vi "LSMcontroller_v64_updatedwaveformhandling.vi"() -> ()   [LabVIEW 2015] (continued)
                                n1313 = case shown="False" w3862 {
                                tunnel: [w3868 w3888] -> w3861
                                tunnel: [w3867 FALSE ("removal")] -> w3860
                                tunnel: [w3866 w3886] -> w3859
                                tunnel: w3858 -> [w3865 _]
                                frame False {
                                n1314 = case shown="False" w3865 {
                                tunnel: [FALSE ("addition") FALSE ("addition")] -> w3868
                                tunnel: [w3870 FALSE ("removal")] -> w3867
                                tunnel: [w3869 _] -> w3866
                                frame False {
                                n1315 = call "configuration.vi"("command"="get") -> ("config out"=w3876:T11)  [unwired: 2 in, 1 out]
                                n1316 = Unbundle By Name(w3876) -> ("2P shutter"=w3873:i32)
                                n1317 = call "2pparameters.vi"("command"="get") -> ("params out"=w3874:T10)  [unwired: 1 in]
                                n1318 = in-place {
                                in-place-border: w3873 -> [w3883]
                                in-place-border: [w3880] -> w3870
                                in-place-border: [w3879] -> w3869
                                n1319 = in-place-cluster #25(w3874) -> ("aDO"=w3882:u32[])
                                n1320 = call "remove channel from active arrayv2.vi"("line array in"=w3882, "line to remove"=w3883) -> ("line array out"=w3881:u32[], "removal"=w3880:bool, "index"=w3879:i32)
                                n1321 = in-place-cluster #25("aDO"=w3881) -> (w3871:T10)
                                }
                                n1322 = call "2pparameters.vi"("Params in"=w3871, "command"="set") -> ()  [unwired: 1 out]
                                }
                                frame True {
                                }
                                }
                                }
                                frame True {
                                n1323 = call "configuration.vi"("command"="get") -> ("config out"=w3890:T11)  [unwired: 2 in, 1 out]
                                n1324 = call "2pparameters.vi"("command"="get") -> ("params out"=w3894:T10)  [unwired: 1 in]
                                n1325 = Unbundle By Name(w3890) -> ("2P shutter"=w3889:i32)
                                n1326 = in-place {
                                in-place-border: w3889 -> [w3900]
                                in-place-border: [w3897] -> w3888
                                in-place-border: [w3896] -> w3886
                                n1327 = in-place-cluster #26(w3894) -> ("aDO"=w3899:u32[])
                                n1328 = call "add channel to active arrayv2.vi"("line array in"=w3899, "line to add"=w3900) -> ("line array out"=w3898:u32[], "addition"=w3897:bool, "index"=w3896:i32)
                                n1329 = in-place-cluster #26("aDO"=w3898) -> (w3892:T10)
                                }
                                n1330 = call "2pparameters.vi"("Params in"=w3892, "command"="set") -> ()  [unwired: 1 out]
                                }
                                }
                                }
                                frame #3 {
                                n1331 = local read "Measurement"() -> (w3904:T4)
                                n1332 = To Unsigned Long Integer(number=w3904) -> (unsigned 32bit integer=w3905:u32)
                                n1333 = case shown="5..7" w3905 {
                                tunnel: [FALSE ("addition") w3923] -> w3903
                                tunnel: [w3908 FALSE ("removal")] -> w3902
                                tunnel: [w3906 w3921] -> w3901
                                frame 0..4, Default {
                                n1334 = call "configuration.vi"("command"="get") -> ("config out"=w3914:T11)  [unwired: 2 in, 1 out]
                                n1335 = Unbundle By Name(w3914) -> ("LT timestamp"=w3911:u32)
                                n1336 = call "2pparameters.vi"("command"="get") -> ("params out"=w3912:T10)  [unwired: 1 in]
                                n1337 = in-place {
                                in-place-border: w3911 -> [w3920]
                                in-place-border: [w3917] -> w3908
                                in-place-border: [w3916] -> w3906
                                n1338 = in-place-cluster #27(w3912) -> ("aDO"=w3919:u32[])
                                n1339 = call "remove channel from active arrayv2.vi"("line array in"=w3919, "line to remove"=w3920) -> ("line array out"=w3918:u32[], "removal"=w3917:bool, "index"=w3916:i32)
                                n1340 = in-place-cluster #27("aDO"=w3918) -> (w3909:T10)
                                }
                                n1341 = call "2pparameters.vi"("Params in"=w3909, "command"="set") -> ()  [unwired: 1 out]
                                }
                                frame 5..7 {
                                n1342 = call "configuration.vi"("command"="get") -> ("config out"=w3929:T11)  [unwired: 2 in, 1 out]
                                n1343 = Unbundle By Name(w3929) -> ("LT timestamp"=w3926:u32)
                                n1344 = call "2pparameters.vi"("command"="get") -> ("params out"=w3927:T10)  [unwired: 1 in]
                                n1345 = in-place {
                                in-place-border: w3926 -> [w3935]
                                in-place-border: [w3932] -> w3923
                                in-place-border: [w3931] -> w3921
                                n1346 = in-place-cluster #28(w3927) -> ("aDO"=w3934:u32[])
                                n1347 = call "add channel to active arrayv2.vi"("line array in"=w3934, "line to add"=w3935) -> ("line array out"=w3933:u32[], "addition"=w3932:bool, "index"=w3931:i32)
                                n1348 = in-place-cluster #28("aDO"=w3933) -> (w3924:T10)
                                }
                                n1349 = call "2pparameters.vi"("Params in"=w3924, "command"="set") -> ()  [unwired: 1 out]
                                }
                                }
                                }
                                }
                                }
                                frame #1 {
                                n1350 = Or(x=w3942, y=w3943) -> (x .or. y?=w3941:bool)
                                n1351 = case shown="True" w3941 {
                                frame False {
                                }
                                frame True {
                                # "update GUI"
                                n1352 = call "Used AO lines.vi"() -> ("used AO names"=w3947:string[], "used AO lines"=w3949:tag[])  [unwired: 2 in]
                                n1353 = control-ref of="Analog Lines Plot"() -> (w3948:refnum<vi>)
                                n1354 = local write "Analog Used Lines"(w3949) -> ()
                                n1355 = local write "Analog Used Names"(w3947) -> ()
                                n1356 = call "prepAOWaveplot.vi"("WaveformGraph in"=w3948, "Analog Used Names"=w3947) -> ()  [unwired: 1 in]
                                }
                                }
                                n1357 = Compound Arithmetic op=OR(w3939, w3938, w3937, w3936) -> (w3940:bool)
                                n1358 = case shown="True" w3940 {
                                frame False {
                                }
                                frame True {
                                n1359 = control-ref of="Digital Lines Plot"() -> (w3944:refnum<vi>)
                                n1360 = call "Used DO lines.vi"() -> ("used DO names"=w3945:string[], "used DO lines"=w3946:tag[])  [unwired: 2 in]
                                n1361 = local write "Digital Used Lines"(w3946) -> ()
                                n1362 = local write "Digital Used Names"(w3945) -> ()
                                n1363 = call "prepDOWaveplot.vi"("DigitalGraph in"=w3944, "used DO names"=w3945) -> ()  [unwired: 1 in]
                                }
                                }
                                }
                                frame #2 {
                                n1364 = case shown="False" w3953 {
                                tunnel: [w3956 w3982] -> w3952
                                tunnel: [w3955 w3980] -> w3951
                                tunnel: [w3954 _] -> w3950
                                frame False {
                                n1365 = stacked-sequence {
                                seq-local: [w3958 _] -> [_ w3973]
                                tunnel: [w3958 _] -> w3956
                                tunnel: [w3961 _] -> w3955
                                tunnel: [w3957 _] -> w3954
                                frame #0 {
                                n1366 = call "configuration.vi"("command"="get") -> ("config out"=w3969:T11)  [unwired: 2 in, 1 out]
                                n1367 = call "waveformparamsv2.vi"("command"="get") -> ("Params out"=w3963:T14)  [unwired: 4 in, 2 out]
                                n1368 = Unbundle By Name(w3969) -> ("Voltage to Xgalvo"=w3970:i32)
                                n1369 = call "2pparameters.vi"("command"="get") -> ("params out"=w3966:T10)  [unwired: 1 in]
                                n1370 = Unbundle By Name(w3963) -> ("AO parameters"=w3962:T15)
                                n1371 = Unbundle By Name(w3966) -> ("aAO"=w3967:u32[])
                                n1372 = call "waveformsAObuffer.vi"("command"="get") -> ("AO wf out"=w3959:waveform(dbl)[])  [unwired: 1 in]
                                n1373 = Search 1D Array(1D array=w3967, element=w3970) -> (index of element=w3958:i32)  [unwired: 1 in]
                                n1374 = Index Array(array=w3959, index=w3958) -> (element=w3957:waveform(dbl))
                                n1375 = Index Array(array=w3962, index=w3958) -> (element=w3961:T16)
                                }
                                frame #1 {
                                w3974 = 0.0 ("Step size (V)")
                                n1376 = local read "Meastab"() -> (w3972:enum32{"X-Y Image", "Linescan", "Timetrace"})
                                n1377 = case shown="\"X-Y Image\", Default" w3972 {
                                tunnel: [w3976 w3977] -> w3971
                                frame "X-Y Image", Default {
                                n1378 = local read "Sampling rate"() -> (w3976:dbl)
                                }
                                frame "Timetrace" {
                                n1379 = local read "srateAODOtt"() -> (w3977:dbl)
                                }
                                }
                                n1380 = call "replace AO XYwfparam.vi"("Baseline (V)"=w3974, "Start amplitude (V)"=w3974, "Cycles"=w3974, "Repeats"=w3974, "index of AO wave"=w3973, "Step size (V)"=w3974, "DC (%)"=w3974, "Sampling frequency (Hz)"=w3971, "Period (ms)"=w3974, "Cycle length (s)"=w3974, "Pulses"=w3974, "padding value"=w3974, "Matlab wave name"=path "xwave") -> ()  [unwired: 3 in]
                                }
                                }
                                }
                                frame True {
                                w3981 = 0.0 ("Repeats")
                                n1381 = local read "Meastab"() -> (w3979:enum32{"X-Y Image", "Linescan", "Timetrace"})
                                n1382 = case shown="\"X-Y Image\", Default" w3979 {
                                tunnel: [w3998 w3999] -> w3978
                                frame "X-Y Image", Default {
                                n1383 = local read "Sampling rate"() -> (w3998:dbl)
                                }
                                frame "Timetrace" {
                                n1384 = local read "srateAODOtt"() -> (w3999:dbl)
                                }
                                }
                                n1385 = call "2pparameters.vi"("command"="get") -> ("params out"=w3984:T10)  [unwired: 1 in]
                                n1386 = call "configuration.vi"("command"="get") -> ("config out"=w3987:T11)  [unwired: 2 in, 1 out]
                                n1387 = call "waveformparamsv2.vi"("command"="get") -> ("Params out"=w3995:T14)  [unwired: 4 in, 2 out]
                                n1388 = Unbundle By Name(w3987) -> ("Voltage to Xgalvo"=w3988:i32)
                                n1389 = Unbundle By Name(w3995) -> ("AO parameters"=w3992:T15)
                                n1390 = Unbundle By Name(w3984) -> ("aAO"=w3985:u32[])
                                n1391 = Search 1D Array(1D array=w3985, element=w3988) -> (index of element=w3982:i32)  [unwired: 1 in]
                                n1392 = Index Array(array=w3992, index=0) -> (element=w3993:T16)
                                n1393 = Bundle By Name(cluster=w3993, "AOtab"=-1.0 ("Repeats"), "Repeats"=w3981, "Cycles"=w3981, "Start amplitude (V)"=w3981, "Baseline (V)"=w3981, "Step size (V)"=w3981, "DC (%)"=w3981, "Sampling frequency (Hz)"=w3978, "Period (ms)"=w3981, "Offset (V)"=w3981, "Amplitude (V)"=w3981, "Frequency"=w3981, "Tri Repeats"=w3981, "phase shift (ms)"=w3981, "Pulses"=w3981, "Matlab wave file"=path "xwave", "padding value"=w3981) -> (w3980:T16)
                                n1394 = Build Array(w3980) -> (w3990:T15)
                                n1395 = call "waveformparamsv2.vi"("command"="add AO", "add AO"=w3990) -> ()  [unwired: 3 in, 3 out]
                                }
                                }
                                }
                                frame #3 {
                                n1396 = case shown="False" w4003 {
                                tunnel: [w4006 w4032] -> w4002
                                tunnel: [w4005 w4030] -> w4001
                                tunnel: [w4004 _] -> w4000
                                frame False {
                                n1397 = stacked-sequence {
                                seq-local: [w4008 _] -> [_ w4023]
                                tunnel: [w4008 _] -> w4006
                                tunnel: [w4011 _] -> w4005
                                tunnel: [w4007 _] -> w4004
                                frame #0 {
                                n1398 = call "configuration.vi"("command"="get") -> ("config out"=w4019:T11)  [unwired: 2 in, 1 out]
                                n1399 = call "waveformparamsv2.vi"("command"="get") -> ("Params out"=w4013:T14)  [unwired: 4 in, 2 out]
                                n1400 = Unbundle By Name(w4019) -> ("Voltage to Ygalvo"=w4020:i32)
                                n1401 = call "2pparameters.vi"("command"="get") -> ("params out"=w4016:T10)  [unwired: 1 in]
                                n1402 = Unbundle By Name(w4013) -> ("AO parameters"=w4012:T15)
                                n1403 = Unbundle By Name(w4016) -> ("aAO"=w4017:u32[])
                                n1404 = call "waveformsAObuffer.vi"("command"="get") -> ("AO wf out"=w4009:waveform(dbl)[])  [unwired: 1 in]
                                n1405 = Search 1D Array(1D array=w4017, element=w4020) -> (index of element=w4008:i32)  [unwired: 1 in]
                                n1406 = Index Array(array=w4009, index=w4008) -> (element=w4007:waveform(dbl))
                                n1407 = Index Array(array=w4012, index=w4008) -> (element=w4011:T16)
                                }
                                frame #1 {
                                w4024 = 0.0 ("Step size (V)")
                                n1408 = local read "Meastab"() -> (w4022:enum32{"X-Y Image", "Linescan", "Timetrace"})
                                n1409 = case shown="\"X-Y Image\", Default" w4022 {
                                tunnel: [w4026 w4027] -> w4021
                                frame "X-Y Image", Default {
                                n1410 = local read "Sampling rate"() -> (w4026:dbl)
                                }
                                frame "Timetrace" {
                                n1411 = local read "srateAODOtt"() -> (w4027:dbl)
                                }
                                }
                                n1412 = call "replace AO XYwfparam.vi"("Baseline (V)"=w4024, "Start amplitude (V)"=w4024, "Cycles"=w4024, "Repeats"=w4024, "index of AO wave"=w4023, "Step size (V)"=w4024, "DC (%)"=w4024, "Sampling frequency (Hz)"=w4021, "Period (ms)"=w4024, "Cycle length (s)"=w4024, "Pulses"=w4024, "padding value"=w4024, "Matlab wave name"=path "ywave") -> ()  [unwired: 3 in]
                                }
                                }
                                }
                                frame True {
                                w4031 = 0.0 ("Repeats")
                                n1413 = local read "Meastab"() -> (w4029:enum32{"X-Y Image", "Linescan", "Timetrace"})
                                n1414 = case shown="\"X-Y Image\", Default" w4029 {
                                tunnel: [w4048 w4049] -> w4028
                                frame "X-Y Image", Default {
                                n1415 = local read "Sampling rate"() -> (w4048:dbl)
                                }
                                frame "Timetrace" {
                                n1416 = local read "srateAODOtt"() -> (w4049:dbl)
                                }
                                }
                                n1417 = call "2pparameters.vi"("command"="get") -> ("params out"=w4034:T10)  [unwired: 1 in]
                                n1418 = call "configuration.vi"("command"="get") -> ("config out"=w4037:T11)  [unwired: 2 in, 1 out]
                                n1419 = call "waveformparamsv2.vi"("command"="get") -> ("Params out"=w4046:T14)  [unwired: 4 in, 2 out]
                                n1420 = Unbundle By Name(w4037) -> ("Voltage to Ygalvo"=w4038:i32)
                                n1421 = Unbundle By Name(w4046) -> ("AO parameters"=w4043:T15)
                                n1422 = Unbundle By Name(w4034) -> ("aAO"=w4035:u32[])
                                n1423 = Search 1D Array(1D array=w4035, element=w4038) -> (index of element=w4032:i32)  [unwired: 1 in]
                                n1424 = Index Array(array=w4043, index=0) -> (element=w4044:T16)
                                n1425 = Bundle By Name(cluster=w4044, "AOtab"=-1.0 ("Repeats"), "Repeats"=w4031, "Cycles"=w4031, "Start amplitude (V)"=w4031, "Baseline (V)"=w4031, "Step size (V)"=w4031, "DC (%)"=w4031, "Sampling frequency (Hz)"=w4028, "Period (ms)"=w4031, "Offset (V)"=w4031, "Amplitude (V)"=w4031, "Frequency"=w4031, "Tri Repeats"=w4031, "phase shift (ms)"=w4031, "Pulses"=w4031, "Matlab wave file"=path "ywave", "padding value"=w4031) -> (w4030:T16)
                                n1426 = Build Array(w4030) -> (w4041:T15)
                                n1427 = call "waveformparamsv2.vi"("command"="add AO", "add AO"=w4041) -> ()  [unwired: 3 in, 3 out]
                                }
                                }
                                }
                                frame #4 {
                                n1428 = call "2pparameters.vi"("command"="get") -> ("params out"=w4055:T10)  [unwired: 1 in]
                                n1429 = Unbundle By Name(w4055) -> ("wavdet"=w4054:bool, "Pel"=w4051:sgl, "refwfsize"=w4050:dbl, "srateAODO"=w4053:sgl)
                                n1430 = case shown="True" w4054 {
                                tunnel: [w4059 w4069] -> w4057
                                tunnel: w4053 -> [w4060 w4071]
                                tunnel: w4051 -> [_ w4067]
                                tunnel: w4050 -> [_ w4066]
                                frame False {
                                n1431 = call "X-array-databuffer.vi"("command"=enum16{"get", "set", "clear", "append"}."get") -> ("array out"=w4063:dbl[])  [unwired: 3 in, 1 out]
                                n1432 = Reciprocal(x=w4060) -> (1/x=w4061:sgl)
                                n1433 = Bundle By Name("Y"=w4063, "dt"=w4061) -> (w4059:waveform(dbl))  [unwired: 1 in]
                                }
                                frame True {
                                n1434 = To Double Precision Float(number=w4067) -> (double precision float=w4068:dbl)
                                n1435 = Divide(x=w4066, y=w4068) -> (x/y=w4065:dbl)
                                n1436 = Round Toward +Infinity(x=w4065) -> (ceil(x): smallest int >= x=w4064:dbl)
                                n1437 = call "X-array-databuffer.vi"("command"=enum16{"get", "set", "clear", "append"}."get") -> ("array out"=w4073:dbl[])  [unwired: 3 in, 1 out]
                                n1438 = Reciprocal(x=w4071) -> (1/x=w4072:sgl)
                                n1439 = for {
                                N: w4064 -> [_]
                                tunnel: w4073 -> [w4075]
                                tunnel: [w4075] -> w4070 mode=concatenating
                                }
                                n1440 = Bundle By Name("Y"=w4070, "dt"=w4072) -> (w4069:waveform(dbl))  [unwired: 1 in]
                                }
                                }
                                n1441 = case shown="True" w4058 {
                                tunnel: w4057 -> [w4077 w4083]
                                tunnel: w4052 -> [w4078 _]
                                frame False {
                                n1442 = call "waveformsAObuffer.vi"("command"="get") -> ("AO wf out"=w4081:waveform(dbl)[])  [unwired: 1 in]
                                n1443 = property on="refwf" class="Ring (strict)" props=["RingText", "Text"]() -> ()  [unwired: 2 in, 3 out]
                                n1444 = Replace Array Subset(array=w4081, new element=w4077, index=w4078) -> (w4076:waveform(dbl)[])
                                n1445 = call "waveformsAObuffer.vi"("AO wf in"=w4076, "command"="set") -> ()  [unwired: 1 out]
                                }
                                frame True {
                                n1446 = call "waveformsAObuffer.vi"("command"="get") -> ("AO wf out"=w4085:waveform(dbl)[])  [unwired: 1 in]
                                n1447 = Build Array (concatenate)(w4085, w4083) -> (w4082:waveform(dbl)[])
                                n1448 = call "waveformsAObuffer.vi"("AO wf in"=w4082, "command"="set") -> ()  [unwired: 1 out]
                                }
                                }
                                }
                                frame #5 {
                                n1449 = call "2pparameters.vi"("command"="get") -> ("params out"=w4097:T10)  [unwired: 1 in]
                                n1450 = Unbundle By Name(w4097) -> ("wavdet"=w4096:bool, "Pel"=w4094:sgl, "refwfsize"=w4095:dbl, "srateAODO"=w4090:sgl)
                                n1451 = To Double Precision Float(number=w4094) -> (double precision float=w4093:dbl)
                                n1452 = Divide(x=w4095, y=w4093) -> (x/y=w4092:dbl)
                                n1453 = Round Toward +Infinity(x=w4092) -> (ceil(x): smallest int >= x=w4091:dbl)
                                n1454 = case shown="True" w4096 {
                                tunnel: [w4101 w4107] -> w4087
                                tunnel: w4091 -> [_ w4104]
                                tunnel: w4090 -> [w4102 w4109]
                                frame False {
                                n1455 = call "Y-array-databuffer.vi"("command"=enum16{"get", "set", "clear", "append"}."get") -> ("array out"=w4099:dbl[])  [unwired: 3 in, 1 out]
                                n1456 = Reciprocal(x=w4102) -> (1/x=w4103:sgl)
                                n1457 = Bundle By Name("Y"=w4099, "dt"=w4103) -> (w4101:waveform(dbl))  [unwired: 1 in]
                                }
                                frame True {
                                n1458 = call "Y-array-databuffer.vi"("command"=enum16{"get", "set", "clear", "append"}."get") -> ("array out"=w4105:dbl[])  [unwired: 3 in, 1 out]
                                n1459 = Reciprocal(x=w4109) -> (1/x=w4110:sgl)
                                n1460 = for {
                                N: w4104 -> [_]
                                tunnel: w4105 -> [w4111]
                                tunnel: [w4111] -> w4108 mode=concatenating
                                }
                                n1461 = Bundle By Name("Y"=w4108, "dt"=w4110) -> (w4107:waveform(dbl))  [unwired: 1 in]
                                }
                                }
                                n1462 = case shown="False" w4089 {
                                tunnel: w4087 -> [w4114 w4119]
                                tunnel: w4088 -> [w4115 _]
                                frame False {
                                n1463 = call "waveformsAObuffer.vi"("command"="get") -> ("AO wf out"=w4117:waveform(dbl)[])  [unwired: 1 in]
                                n1464 = Replace Array Subset(array=w4117, new element=w4114, index=w4115) -> (w4112:waveform(dbl)[])
                                n1465 = call "waveformsAObuffer.vi"("AO wf in"=w4112, "command"="set") -> ()  [unwired: 1 out]
                                }
                                frame True {
                                n1466 = call "waveformsAObuffer.vi"("command"="get") -> ("AO wf out"=w4121:waveform(dbl)[])  [unwired: 1 in]
                                n1467 = Build Array (concatenate)(w4121, w4119) -> (w4118:waveform(dbl)[])
                                n1468 = call "waveformsAObuffer.vi"("AO wf in"=w4118, "command"="set") -> ()  [unwired: 1 out]
                                }
                                }
                                }
                                frame #6 {
                                n1469 = Build Array(w4126, w4125) -> (w4129:bool[])
                                n1470 = Boolean Array To Number(Boolean array=w4129) -> (number=w4128:u32)
                                n1471 = case shown="2" w4128 {
                                tunnel: w4127 -> [_ _ _ _]
                                tunnel: w4124 -> [_ w4152 _ w4165]
                                tunnel: [_ w4151 _ w4162] -> w4123
                                frame 1 {
                                w4139 = 0.0 ("DOtab")
                                n1472 = call "2pparameters.vi"("command"="get") -> ("params out"=w4136:T10)  [unwired: 1 in]
                                n1473 = call "waveformparamsv2.vi"("command"="get") -> ("Params out"=w4147:T14)  [unwired: 4 in, 2 out]
                                n1474 = Unbundle By Name(w4147) -> ("DO parameters"=w4145:T17)
                                n1475 = Unbundle By Name(w4136) -> ("srate"=w4132:sgl, "Pel"=w4135:sgl)
                                n1476 = To Double Precision Float(number=w4132) -> (double precision float=w4130:dbl)
                                n1477 = To Double Precision Float(number=w4132) -> (double precision float=w4131:dbl)
                                n1478 = To Double Precision Float(number=w4135) -> (double precision float=w4134:dbl)
                                n1479 = Divide(x=w4131, y=w4134) -> (x/y=w4133:dbl)
                                n1480 = Index Array(array=w4145, index=0) -> (element=w4144:T18)
                                n1481 = Bundle By Name(cluster=w4144, "Digital DC (%)"=100.0, "Digital phase"=w4139, "Digital Freq (Hz)"=w4133, "Sampling frequency (Hz)"=w4130, "Digital time offset (s)"=w4139, "padding value"=0.0, "matlab wave file"=path "2Pshutter", "DOtab"=0.0) -> (w4142:T18)
                                n1482 = Build Array(w4142) -> (w4141:T17)
                                n1483 = call "waveformparamsv2.vi"("command"="add DO", "add DO"=w4141) -> ()  [unwired: 3 in, 3 out]
                                }
                                frame 2 {
                                n1484 = call "waveformparamsv2.vi"("command"="get") -> ("Params out"=w4154:T14)  [unwired: 4 in, 2 out]
                                n1485 = in-place {
                                in-place-border: w4152 -> [w4158]
                                in-place-border: [w4157] -> w4151
                                n1486 = in-place-cluster #29(w4154) -> ("DO parameters"=w4160:T17)
                                n1487 = Delete From Array(array=w4160, length=1, index=w4158) -> (deleted portion=w4157:T17, array with subset deleted=w4159:T17)
                                n1488 = in-place-cluster #29("DO parameters"=w4159) -> (w4153:T14)
                                }
                                n1489 = call "waveformparamsv2.vi"("command"="set", "Params in"=w4153) -> ()  [unwired: 3 in, 3 out]
                                }
                                frame 3, Default {
                                }
                                frame 0 {
                                n1490 = call "2pparameters.vi"("command"="get") -> ("params out"=w4167:T10)  [unwired: 1 in]
                                n1491 = Unbundle By Name(w4167) -> ("wavdet"=w4164:bool, "autoshutter"=w4166:bool)
                                n1492 = case shown="True" w4166 {
                                tunnel: w4165 -> [_ w4171]
                                tunnel: w4164 -> [_ w4170]
                                tunnel: [_ w4169] -> w4163
                                frame False {
                                }
                                frame True {
                                n1493 = case shown="False" w4170 {
                                tunnel: w4171 -> [w4173 _]
                                tunnel: [w4172 _] -> w4169
                                frame False {
                                n1494 = stacked-sequence {
                                tunnel: w4173 -> [w4175 w4189]
                                tunnel: [w4174 _] -> w4172
                                frame #0 {
                                n1495 = call "waveformparamsv2.vi"("command"="get") -> ("Params out"=w4177:T14)  [unwired: 4 in, 2 out]
                                n1496 = Unbundle By Name(w4177) -> ("DO parameters"=w4176:T17)
                                n1497 = Index Array(array=w4176, index=w4175) -> (element=w4174:T18)
                                }
                                frame #1 {
                                w4188 = 0.0 ("padding value")
                                n1498 = call "2pparameters.vi"("command"="get") -> ("params out"=w4186:T10)  [unwired: 1 in]
                                n1499 = Unbundle By Name(w4186) -> ("srate"=w4183:sgl, "Pel"=w4185:sgl)
                                n1500 = To Double Precision Float(number=w4183) -> (double precision float=w4181:dbl)
                                n1501 = To Double Precision Float(number=w4183) -> (double precision float=w4182:dbl)
                                n1502 = To Double Precision Float(number=w4185) -> (double precision float=w4184:dbl)
                                n1503 = Divide(x=w4182, y=w4184) -> (x/y=w4180:dbl)
                                n1504 = call "replace DO wf param.vi"("Digital Freq (Hz)"=w4180, "Digital DC (%)"=100.0, "Digital phase"=w4188, "Sampling frequency (Hz)"=w4181, "Digital time offset (s)"=w4188, "index of DO wave"=w4189, "padding value"=w4188, "matlab wave file"=path "2Pshutter" ("matlab wave number")) -> ()  [unwired: 3 in]
                                }
                                }
                                }
                                frame True {
                                }
                                }
                                }
                                }
                                n1505 = Build Array(w4163) -> (w4162:T17)
                                }
                                }
                                }
                                frame #7 {
                                n1506 = Build Array(w4194, w4193) -> (w4196:bool[])
                                n1507 = Boolean Array To Number(Boolean array=w4196) -> (number=w4195:u32)
                                n1508 = case shown="0" w4195 {
                                tunnel: w4192 -> [_ w4238 _ w4245]
                                tunnel: [_ w4237 _ w4243] -> w4191
                                frame 1 {
                                n1509 = call "2pparameters.vi"("command"="get") -> ("params out"=w4203:T10)  [unwired: 1 in]
                                n1510 = Unbundle By Name(w4203) -> ("wavdet"=w4204:bool, "Pel"=w4206:sgl, "refwfsize"=w4207:dbl, "srateAODO"=w4205:sgl)
                                n1511 = call "waveformsDObuffer.vi"("command"="get") -> ("DO wf out"=w4199:digitalwaveform[])  [unwired: 1 in]
                                n1512 = case shown="False" w4204 {
                                tunnel: [w4212 w4222] -> w4201
                                tunnel: w4205 -> [w4217 w4233]
                                tunnel: w4206 -> [w4211 w4226]
                                tunnel: w4207 -> [_ w4230]
                                frame False {
                                w4215 = u16 0 items=["unsigned binary", "offset binary", "2's complement"] ("data format (offset binary)")
                                n1513 = Initialize Array(sgl 1.0, w4211) -> (w4208:sgl[])
                                n1514 = Reciprocal(x=w4217) -> (1/x=w4218:sgl)
                                n1515 = Bundle By Name("Y"=w4208, "dt"=w4218) -> (w4213:waveform(sgl))  [unwired: 1 in]
                                n1516 = call-poly <vilib>:"Analog to Digital.vi"("data format (offset binary)"=w4215, "compress digital (T)"=TRUE, "full-scale range (pk-pk)"=1.0, "resolution (16 bit)"=1, "analog waveform"=w4213) -> ("digital waveform"=w4212:digitalwaveform)  [unwired: 3 in, 3 out]
                                }
                                frame True {
                                w4225 = u16 0 items=["unsigned binary", "offset binary", "2's complement"] ("data format (offset binary)")
                                n1517 = To Double Precision Float(number=w4226) -> (double precision float=w4231:dbl)
                                n1518 = Initialize Array(sgl 1.0, w4226) -> (w4219:sgl[])
                                n1519 = Divide(x=w4230, y=w4231) -> (x/y=w4228:dbl)
                                n1520 = Round Toward +Infinity(x=w4228) -> (ceil(x): smallest int >= x=w4229:dbl)
                                n1521 = for {
                                N: w4229 -> [_]
                                tunnel: w4219 -> [w4235]
                                tunnel: [w4235] -> w4232 mode=concatenating
                                }
                                n1522 = Reciprocal(x=w4233) -> (1/x=w4234:sgl)
                                n1523 = Bundle By Name("Y"=w4232, "dt"=w4234) -> (w4223:waveform(sgl))  [unwired: 1 in]
                                n1524 = call-poly <vilib>:"Analog to Digital.vi"("data format (offset binary)"=w4225, "compress digital (T)"=TRUE, "full-scale range (pk-pk)"=1.0, "resolution (16 bit)"=1, "analog waveform"=w4223) -> ("digital waveform"=w4222:digitalwaveform)  [unwired: 3 in, 3 out]
                                }
                                }
                                n1525 = Build Array (concatenate)(w4199, w4201) -> (w4197:digitalwaveform[])
                                n1526 = call "waveformsDObuffer.vi"("DO wf in"=w4197, "command"="set") -> ()  [unwired: 1 out]
                                }
                                frame 2 {
                                n1527 = call "waveformsDObuffer.vi"("command"="get") -> ("DO wf out"=w4240:digitalwaveform[])  [unwired: 1 in]
                                n1528 = Delete From Array(array=w4240, length=1, index=w4238) -> (deleted portion=w4237:digitalwaveform[], array with subset deleted=w4236:digitalwaveform[])
                                n1529 = call "waveformsDObuffer.vi"("DO wf in"=w4236, "command"="set") -> ()  [unwired: 1 out]
                                }
                                frame 3, Default {
                                }
                                frame 0 {
                                n1530 = call "2pparameters.vi"("command"="get") -> ("params out"=w4247:T10)  [unwired: 1 in]
                                n1531 = Unbundle By Name(w4247) -> ("autoshutter"=w4246:bool, "wavdet"=w4244:bool)
                                n1532 = case shown="True" w4246 {
                                tunnel: w4245 -> [_ w4251]
                                tunnel: w4244 -> [_ w4250]
                                tunnel: [_ w4249] -> w4243
                                frame False {
                                }
                                frame True {
                                n1533 = case shown="False" w4250 {
                                tunnel: w4251 -> [w4255 _]
                                tunnel: [w4253 _] -> w4249
                                frame False {
                                w4262 = u16 0 items=["unsigned binary", "offset binary", "2's complement"] ("data format (offset binary)")
                                n1534 = call "2pparameters.vi"("command"="get") -> ("params out"=w4269:T10)  [unwired: 1 in]
                                n1535 = call "waveformsDObuffer.vi"("command"="get") -> ("DO wf out"=w4256:digitalwaveform[])  [unwired: 1 in]
                                n1536 = Unbundle By Name(w4269) -> ("Pel"=w4271:sgl, "srate"=w4270:sgl)
                                n1537 = Index Array(array=w4256, index=w4255) -> (element=w4254:digitalwaveform)
                                n1538 = Build Array(w4254) -> (w4253:digitalwaveform[])
                                n1539 = Initialize Array(sgl 1.0, w4271) -> (w4257:sgl[])
                                n1540 = Reciprocal(x=w4270) -> (1/x=w4264:sgl)
                                n1541 = Bundle By Name("Y"=w4257, "dt"=w4264) -> (w4260:waveform(sgl))  [unwired: 1 in]
                                n1542 = call-poly <vilib>:"Analog to Digital.vi"("data format (offset binary)"=w4262, "compress digital (T)"=TRUE, "full-scale range (pk-pk)"=1.0, "resolution (16 bit)"=1, "analog waveform"=w4260) -> ("digital waveform"=w4267:digitalwaveform)  [unwired: 3 in, 3 out]
                                n1543 = Replace Array Subset(array=w4256, new element=w4267, index=w4255) -> (w4252:digitalwaveform[])
                                n1544 = call "waveformsDObuffer.vi"("DO wf in"=w4252, "command"="set") -> ()  [unwired: 1 out]
                                }
                                frame True {
                                }
                                }
                                }
                                }
                                }
                                }
                                }
                                frame #8 {
                                n1545 = Build Array(w4275, w4274) -> (w4277:bool[])
                                n1546 = Boolean Array To Number(Boolean array=w4277) -> (number=w4276:u32)
                                n1547 = case shown="0" w4276 {
                                tunnel: w4273 -> [_ w4303 _ w4315]
                                tunnel: [_ w4302 _ w4313] -> w4272
                                frame 1 {
                                w4290 = 0.0 ("DOtab")
                                n1548 = call "2pparameters.vi"("command"="get") -> ("params out"=w4288:T10)  [unwired: 1 in]
                                n1549 = call "waveformparamsv2.vi"("command"="get") -> ("Params out"=w4298:T14)  [unwired: 4 in, 2 out]
                                n1550 = Unbundle By Name(w4298) -> ("DO parameters"=w4296:T17)
                                n1551 = Unbundle By Name(w4288) -> ("srate"=w4285:sgl, "Pel"=w4287:sgl)
                                n1552 = To Double Precision Float(number=w4285) -> (double precision float=w4283:dbl)
                                n1553 = To Double Precision Float(number=w4285) -> (double precision float=w4284:dbl)
                                n1554 = To Double Precision Float(number=w4287) -> (double precision float=w4279:dbl)
                                n1555 = Divide(x=w4284, y=w4279) -> (x/y=w4286:dbl)
                                n1556 = Index Array(array=w4296, index=0) -> (element=w4295:T18)
                                n1557 = Divide(x=1.0 ("Digital DC (%)"), y=w4279) -> (x/y=w4281:dbl)
                                n1558 = Multiply(x=100.0, y=w4281) -> (x*y=w4278:dbl)
                                n1559 = Bundle By Name(cluster=w4295, "Digital DC (%)"=w4278, "Digital phase"=w4290, "Digital Freq (Hz)"=w4286, "Sampling frequency (Hz)"=w4283, "Digital time offset (s)"=w4290, "padding value"=0.0, "matlab wave file"=path "LT", "DOtab"=0.0) -> (w4293:T18)
                                n1560 = Build Array(w4293) -> (w4292:T17)
                                n1561 = call "waveformparamsv2.vi"("command"="add DO", "add DO"=w4292) -> ()  [unwired: 3 in, 3 out]
                                }
                                frame 2 {
                                n1562 = call "waveformparamsv2.vi"("command"="get") -> ("Params out"=w4305:T14)  [unwired: 4 in, 2 out]
                                n1563 = in-place {
                                in-place-border: w4303 -> [w4309]
                                in-place-border: [w4308] -> w4302
                                n1564 = in-place-cluster #30(w4305) -> ("DO parameters"=w4311:T17)
                                n1565 = Delete From Array(array=w4311, length=1, index=w4309) -> (deleted portion=w4308:T17, array with subset deleted=w4310:T17)
                                n1566 = in-place-cluster #30("DO parameters"=w4310) -> (w4304:T14)
                                }
                                n1567 = call "waveformparamsv2.vi"("command"="set", "Params in"=w4304) -> ()  [unwired: 3 in, 3 out]
                                }
                                frame 3, Default {
                                }
                                frame 0 {
                                n1568 = local read "Measurement"() -> (w4317:T4)
                                n1569 = To Unsigned Long Integer(number=w4317) -> (unsigned 32bit integer=w4316:u32)
                                n1570 = case shown="5..7" w4316 {
                                tunnel: w4315 -> [_ w4319]
                                tunnel: [_ w4318] -> w4314
                                frame 0..4, Default {
                                }
                                frame 5..7 {
                                n1571 = stacked-sequence {
                                tunnel: w4319 -> [w4321 w4330]
                                tunnel: [w4320 _] -> w4318
                                frame #0 {
                                n1572 = call "waveformparamsv2.vi"("command"="get") -> ("Params out"=w4323:T14)  [unwired: 4 in, 2 out]
                                n1573 = Unbundle By Name(w4323) -> ("DO parameters"=w4324:T17)
                                n1574 = Index Array(array=w4324, index=w4321) -> (element=w4320:T18)
                                }
                                frame #1 {
                                w4338 = 0.0 ("padding value")
                                n1575 = call "2pparameters.vi"("command"="get") -> ("params out"=w4336:T10)  [unwired: 1 in]
                                n1576 = Unbundle By Name(w4336) -> ("srate"=w4334:sgl, "Pel"=w4335:sgl)
                                n1577 = To Double Precision Float(number=w4334) -> (double precision float=w4332:dbl)
                                n1578 = To Double Precision Float(number=w4334) -> (double precision float=w4333:dbl)
                                n1579 = To Double Precision Float(number=w4335) -> (double precision float=w4328:dbl)
                                n1580 = Divide(x=1.0 ("Digital DC (%)"), y=w4328) -> (x/y=w4327:dbl)
                                n1581 = Multiply(x=100.0, y=w4327) -> (x*y=w4326:dbl)
                                n1582 = Divide(x=w4333, y=w4328) -> (x/y=w4331:dbl)
                                n1583 = call "replace DO wf param.vi"("Digital Freq (Hz)"=w4331, "Digital DC (%)"=w4326, "Digital phase"=w4338, "Sampling frequency (Hz)"=w4332, "Digital time offset (s)"=w4338, "index of DO wave"=w4330, "padding value"=w4338, "matlab wave file"=path "LT" ("matlab wave number")) -> ()  [unwired: 3 in]
                                }
                                }
                                }
                                }
                                n1584 = Build Array(w4314) -> (w4313:T17)
                                }
                                }
                                }
                                frame #9 {
                                n1585 = Build Array(w4343, w4342) -> (w4345:bool[])
                                n1586 = Boolean Array To Number(Boolean array=w4345) -> (number=w4344:u32)
                                n1587 = case shown="0" w4344 {
                                tunnel: w4341 -> [_ w4397 _ w4401]
                                tunnel: [_ w4392 _ w4398] -> w4340
                                frame 1 {
                                n1588 = call "2pparameters.vi"("command"="get") -> ("params out"=w4352:T10)  [unwired: 1 in]
                                n1589 = Unbundle By Name(w4352) -> ("wavdet"=w4353:bool, "Pel"=w4355:sgl, "refwfsize"=w4356:dbl, "Pel"=w4354:sgl)
                                n1590 = call "waveformsDObuffer.vi"("command"="get") -> ("DO wf out"=w4348:digitalwaveform[])  [unwired: 1 in]
                                n1591 = case shown="True" w4353 {
                                tunnel: [w4360 w4373] -> w4350
                                tunnel: w4354 -> [w4369 w4388]
                                tunnel: w4355 -> [w4359 w4379]
                                tunnel: w4356 -> [_ w4385]
                                frame False {
                                w4363 = u16 0 items=["unsigned binary", "offset binary", "2's complement"] ("data format (offset binary)")
                                n1592 = Initialize Array(sgl 0.0, w4359) -> (w4366:sgl[])
                                n1593 = Replace Array Subset(array=w4366, new element=sgl 1.0, index=0) -> (w4364:sgl[])
                                n1594 = Reciprocal(x=w4369) -> (1/x=w4370:sgl)
                                n1595 = Bundle By Name("Y"=w4364, "dt"=w4370) -> (w4361:waveform(sgl))  [unwired: 1 in]
                                n1596 = call-poly <vilib>:"Analog to Digital.vi"("data format (offset binary)"=w4363, "compress digital (T)"=TRUE, "full-scale range (pk-pk)"=1.0, "resolution (16 bit)"=1, "analog waveform"=w4361) -> ("digital waveform"=w4360:digitalwaveform)  [unwired: 3 in, 3 out]
                                }
                                frame True {
                                w4376 = u16 0 items=["unsigned binary", "offset binary", "2's complement"] ("data format (offset binary)")
                                n1597 = To Double Precision Float(number=w4379) -> (double precision float=w4386:dbl)
                                n1598 = Initialize Array(sgl 0.0, w4379) -> (w4381:sgl[])
                                n1599 = Divide(x=w4385, y=w4386) -> (x/y=w4383:dbl)
                                n1600 = Round Toward +Infinity(x=w4383) -> (ceil(x): smallest int >= x=w4384:dbl)
                                n1601 = Replace Array Subset(array=w4381, new element=sgl 1.0, index=0) -> (w4378:sgl[])
                                n1602 = for {
                                N: w4384 -> [_]
                                tunnel: w4378 -> [w4390]
                                tunnel: [w4390] -> w4387 mode=concatenating
                                }
                                n1603 = Reciprocal(x=w4388) -> (1/x=w4389:sgl)
                                n1604 = Bundle By Name("Y"=w4387, "dt"=w4389) -> (w4374:waveform(sgl))  [unwired: 1 in]
                                n1605 = call-poly <vilib>:"Analog to Digital.vi"("data format (offset binary)"=w4376, "compress digital (T)"=TRUE, "full-scale range (pk-pk)"=1.0, "resolution (16 bit)"=1, "analog waveform"=w4374) -> ("digital waveform"=w4373:digitalwaveform)  [unwired: 3 in, 3 out]
                                }
                                }
                                n1606 = Build Array (concatenate)(w4348, w4350) -> (w4346:digitalwaveform[])
                                n1607 = call "waveformsDObuffer.vi"("DO wf in"=w4346, "command"="set") -> ()  [unwired: 1 out]
                                }
                                frame 2 {
                                n1608 = call "waveformsDObuffer.vi"("command"="get") -> ("DO wf out"=w4394:digitalwaveform[])  [unwired: 1 in]
                                n1609 = Delete From Array(array=w4394, length=1, index=w4397) -> (deleted portion=w4392:digitalwaveform[], array with subset deleted=w4391:digitalwaveform[])
                                n1610 = call "waveformsDObuffer.vi"("DO wf in"=w4391, "command"="set") -> ()  [unwired: 1 out]
                                }
                                frame 3, Default {
                                }
                                frame 0 {
                                n1611 = local read "Measurement"() -> (w4400:T4)
                                n1612 = To Unsigned Long Integer(number=w4400) -> (unsigned 32bit integer=w4399:u32)
                                n1613 = case shown="5..7" w4399 {
                                tunnel: w4401 -> [_ w4404]
                                tunnel: [_ w4403] -> w4398
                                frame 0..4, Default {
                                }
                                frame 5..7 {
                                n1614 = call "2pparameters.vi"("command"="get") -> ("params out"=w4411:T10)  [unwired: 1 in]
                                n1615 = Unbundle By Name(w4411) -> ("wavdet"=w4412:bool, "Pel"=w4414:sgl, "refwfsize"=w4415:dbl, "srateAODO"=w4413:sgl)
                                n1616 = call "waveformsDObuffer.vi"("command"="get") -> ("DO wf out"=w4405:digitalwaveform[])  [unwired: 1 in]
                                n1617 = Index Array(array=w4405, index=w4404) -> (element=w4406:digitalwaveform)
                                n1618 = case shown="True" w4412 {
                                tunnel: [w4419 w4432] -> w4409
                                tunnel: w4413 -> [w4428 w4447]
                                tunnel: w4414 -> [w4418 w4438]
                                tunnel: w4415 -> [_ w4444]
                                frame False {
                                w4422 = u16 0 items=["unsigned binary", "offset binary", "2's complement"] ("data format (offset binary)")
                                n1619 = Initialize Array(sgl 0.0, w4418) -> (w4425:sgl[])
                                n1620 = Replace Array Subset(array=w4425, new element=sgl 1.0, index=0) -> (w4423:sgl[])
                                n1621 = Reciprocal(x=w4428) -> (1/x=w4429:sgl)
                                n1622 = Bundle By Name("Y"=w4423, "dt"=w4429) -> (w4420:waveform(sgl))  [unwired: 1 in]
                                n1623 = call-poly <vilib>:"Analog to Digital.vi"("data format (offset binary)"=w4422, "compress digital (T)"=TRUE, "full-scale range (pk-pk)"=1.0, "resolution (16 bit)"=1, "analog waveform"=w4420) -> ("digital waveform"=w4419:digitalwaveform)  [unwired: 3 in, 3 out]
                                }
                                frame True {
                                w4435 = u16 0 items=["unsigned binary", "offset binary", "2's complement"] ("data format (offset binary)")
                                n1624 = To Double Precision Float(number=w4438) -> (double precision float=w4445:dbl)
                                n1625 = Initialize Array(sgl 0.0, w4438) -> (w4440:sgl[])
                                n1626 = Divide(x=w4444, y=w4445) -> (x/y=w4442:dbl)
                                n1627 = Round Toward +Infinity(x=w4442) -> (ceil(x): smallest int >= x=w4443:dbl)
                                n1628 = Replace Array Subset(array=w4440, new element=sgl 1.0, index=0) -> (w4437:sgl[])
                                n1629 = for {
                                N: w4443 -> [_]
                                tunnel: w4437 -> [w4449]
                                tunnel: [w4449] -> w4446 mode=concatenating
                                }
                                n1630 = Reciprocal(x=w4447) -> (1/x=w4448:sgl)
                                n1631 = Bundle By Name("Y"=w4446, "dt"=w4448) -> (w4433:waveform(sgl))  [unwired: 1 in]
                                n1632 = call-poly <vilib>:"Analog to Digital.vi"("data format (offset binary)"=w4435, "compress digital (T)"=TRUE, "full-scale range (pk-pk)"=1.0, "resolution (16 bit)"=1, "analog waveform"=w4433) -> ("digital waveform"=w4432:digitalwaveform)  [unwired: 3 in, 3 out]
                                }
                                }
                                n1633 = Build Array(w4406) -> (w4403:digitalwaveform[])
                                n1634 = Replace Array Subset(array=w4405, new element=w4409, index=w4404) -> (w4402:digitalwaveform[])
                                n1635 = call "waveformsDObuffer.vi"("DO wf in"=w4402, "command"="set") -> ()  [unwired: 1 out]
                                }
                                }
                                }
                                }
                                }
                                frame #10 {
                                n1636 = local read "Meastab"() -> (w4463:enum32{"X-Y Image", "Linescan", "Timetrace"})
                                n1637 = property on="refwf" class="Ring (strict)"() -> ("RingText.Text"=w4460:string)  [unwired: 2 in, 2 out]
                                n1638 = case shown="\"Timetrace\"" w4463 {
                                tunnel: [w4465 w4466] -> w4464
                                frame "X-Y Image", Default {
                                n1639 = local read "Sampling rate"() -> (w4465:dbl)
                                }
                                frame "Timetrace" {
                                n1640 = local read "srateAODOtt"() -> (w4466:dbl)
                                }
                                }
                                n1641 = call "waveformsAObuffer.vi"("command"="get") -> ("AO wf out"=w4453:waveform(dbl)[])  [unwired: 1 in]
                                n1642 = local read "wavdet"() -> (w4461:bool)
                                n1643 = call "waveformsDObuffer.vi"("command"="get") -> ("DO wf out"=w4457:digitalwaveform[])  [unwired: 1 in]
                                n1644 = call "correctwaveformsizetemp.vi"("new sampling frequency (Hz)"=w4464, "start"=TRUE, "reference waveforms to"=w4460, "Analog waveforms in"=w4453, "stop"=FALSE, "Digital waveforms in"=w4457) -> ("analog wf out"=w4459:waveform(dbl)[], "Digital wf out"=w4452:digitalwaveform[], "measpoints"=w4462:i32)
                                n1645 = call "waveformsDObuffer.vi"("DO wf in"=w4452, "command"="set") -> ()  [unwired: 1 out]
                                n1646 = call "waveformsAObuffer.vi"("AO wf in"=w4459, "command"="set") -> ()  [unwired: 1 out]
                                n1647 = case shown="True" w4461 {
                                tunnel: w4462 -> [_ w4469]
                                tunnel: w4452 -> [_ w4467]
                                frame False {
                                }
                                frame True {
                                n1648 = local write "# of frames"(w4469) -> ()
                                n1649 = call "GetNumCamFramesv2.vi"("Digital Waveform Graph"=w4467) -> ("Numeric"=w4468:i32)  [unwired: 10 in]
                                n1650 = local write "Total Camera Frames"(w4468) -> ()
                                }
                                }
                                }
                                }
                              }
                              frame #7 {
                                # "Disabled for conversion to 64 bit"
                                n1651 = disable-structure shown="Disabled" {
                                frame Disabled {
                                n1652 = local read "Measurement"() -> (w4471:T4)
                                n1653 = case shown="\"Lifetime (scan)\"" w4471 {
                                frame "X-Y-t movie", Default {
                                }
                                frame "Lifetime (scan)" {
                                # "total acquisition time"
                                n1654 = call "2pparameters.vi"("command"="get") -> ("params out"=w4479:T10)  [unwired: 1 in]
                                n1655 = Unbundle By Name(w4479) -> ("measpoints"=w4473:i32, "srateAODO"=w4494:sgl)
                                n1656 = Divide(x=w4473, y=w4494) -> (x/y=w4472:sgl)
                                n1657 = local read "min phot"() -> (w4489:u32)
                                n1658 = local read "expected c/s"() -> (w4490:dbl)
                                n1659 = Multiply(x=w4472, y=1000.0) -> (x*y=w4482:dbl)
                                n1660 = local read "Ch1 ZeroX"() -> (w4487:i32)
                                n1661 = local read "truncate"() -> (w4488:u32)
                                n1662 = To Long Integer(number=w4482) -> (32bit integer=w4491:i32)
                                n1663 = To Long Integer(number=w4490) -> (32bit integer=w4492:i32)
                                n1664 = local read "Number of Bins"() -> (w4483:u32)
                                n1665 = local read "Ch1 Level"() -> (w4485:i32)
                                n1666 = local read "Ch0 ZeroX"() -> (w4486:i32)
                                n1667 = local write "Acquisition time"(w4491) -> ()
                                n1668 = local read "Ch0 Level"() -> (w4484:i32)
                                n1669 = call "lifetimeparameters.vi"("command"="get") -> ("Params out"=w4477:T19)  [unwired: 1 in]
                                n1670 = Add(x=100, y=w4491) -> (x+y=w4481:i32)
                                n1671 = Bundle By Name(cluster=w4477, "acq time"=w4481, "acq rate"=w4492, "# bins"=w4483, "Ch0 Level"=w4484, "Ch1 Level"=w4485, "Ch0 ZeroX"=w4486, "Ch1 ZeroX"=w4487, "min photons"=w4489, "truncate"=w4488) -> (w4476:T19)
                                n1672 = local write "Acquisition rate"(w4492) -> ()
                                n1673 = call "lifetimeparameters.vi"("Params in"=w4476, "command"="set") -> ()  [unwired: 1 out]
                                }
                                }
                                }
                                frame Enabled {
                                }
                                }
                                n1674 = local write "64bit disabled"(TRUE ("64bit disabled")) -> ()
                              }
                              frame #8 {
                                n1675 = call "2pparameters.vi"("command"="get") -> ("params out"=w4505:T10)  [unwired: 1 in]
                                n1676 = Unbundle By Name(w4505) -> ("refreshbuffer"=w4503:i32, "srate"=w4504:sgl)
                                n1677 = local read "wavdet"() -> (w4495:bool)
                                n1678 = To Double Precision Float(number=w4504) -> (double precision float=w4507:dbl)
                                n1679 = To Double Precision Float(number=w4503) -> (double precision float=w4498:dbl)
                                n1680 = case shown="False" w4495 {
                                tunnel: [w4512 w4513] -> w4497
                                frame False {
                                w4512 = 10123 items=["Finite Samples"=10178, "Continuous Samples"=10123, "Hardware Timed Single Point"=12522] ("sample mode")
                                }
                                frame True {
                                w4513 = 10123 items=["Finite Samples"=10178, "Continuous Samples"=10123, "Hardware Timed Single Point"=12522] ("sample mode")
                                }
                                }
                                n1681 = Divide(x=w4498, y=w4507) -> (x/y=w4511:dbl)
                                n1682 = Multiply(x=w4511, y=2.0) -> (x*y=w4508:dbl)
                                n1683 = Max & Min(x=w4508, y=10.0) -> (max(x,y)=w4499:dbl)  [unwired: 1 out]
                                n1684 = call "2pparameters.vi"("command"="get") -> ("params out"=w4502:T10)  [unwired: 1 in]
                                n1685 = Bundle By Name(cluster=w4502, "timeout"=w4499, "sample mode"=w4497) -> (w4500:T10)
                                n1686 = call "2pparameters.vi"("Params in"=w4500, "command"="set") -> ()  [unwired: 1 out]
                              }
                            }
                          }
                          frame #1 {
                            # "Disabled for conversion to 64 bit"
                            n1687 = call "prepAO_img.vi"() -> ("Terminal Name with Device Prefix"=w4515:tag)
                            n1688 = call "prepDO_img.vi"() -> ()  [unwired: 2 in]
                            n1689 = call "prepAI_img.vi"("triggersource"=w4515) -> ()  [unwired: 2 in]
                            n1690 = call "prepCI_img.vi"("ArmStart.DigEdge.Src"=w4515) -> ()  [unwired: 1 in]
                            n1691 = disable-structure shown="Disabled" {
                              frame Disabled {
                                n1692 = local read "Measurement"() -> (w4516:T4)
                                n1693 = case shown="\"Lifetime (contour)\"" w4516 {
                                frame "X-Y-t movie", Default {
                                }
                                frame "Lifetime (contour)" {
                                n1694 = stacked-sequence {
                                frame #0 {
                                n1695 = call "PH-temp.vi"("String"="clear" ("command")) -> ()  [unwired: 2 in, 2 out]
                                n1696 = call "PH-temp-raw.vi"("command"="empty") -> ()  [unwired: 1 in, 1 out]
                                }
                                frame #1 {
                                n1697 = call "calib.vi"() -> ()  [unwired: 1 in]
                                }
                                frame #2 {
                                n1698 = call "setup.vi"() -> ()  [unwired: 1 in]
                                }
                                }
                                }
                                }
                              }
                              frame Enabled {
                              }
                            }
